vi "pid_coef_conv.vi"(11 "PID Control input":T1) -> (3 "PID Control output":T1)   [LabVIEW 2015, in "Hardware.lvlib"]
uses:
  Hardware.lvlib
  Settings/PID Compensator.ctl
  Settings/Settings.lvlib
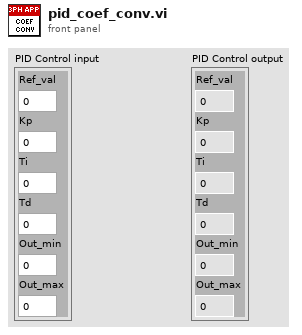
[diagram p1: front panel]
types:
  T1 = typedef "Settings.lvlib/PID Compensator.ctl" = cluster{"Ref_val":sgl, "Kp":sgl, "Ti":sgl, "Td":sgl, "Out_min":sgl, "Out_max":sgl}
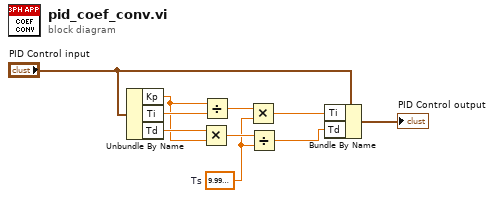
[diagram p0: block diagram]
diagram:
  w3 = sgl 1e-05  # Ts
  n1 = Unbundle By Name("PID Control input") -> ("Kp"=w6:sgl, "Ti"=w7:sgl, "Td"=w8:sgl)
  n2 = Multiply(x=w8, y=w6) -> (x*y=w4:sgl)
  n3 = Divide(x=w6, y=w7) -> (x/y=w5:sgl)
  n4 = Multiply(x=w5, y=w3) -> (x*y=w2:sgl)
  n5 = Divide(x=w4, y=w3) -> (x/y=w1:sgl)
  n6 = Bundle By Name(cluster="PID Control input", "Ti"=w2, "Td"=w1) -> (→"PID Control output":T1)
